vi "Time.Inline Calculate Duration Secs.vi"(8 "Error In Bot":errorcluster, 9 "Start(Sec)":dbl, 11 "Error In Top":errorcluster) -> (0 "Error Out Bot":errorcluster, 1 "Duration(s)":dbl, 3 "Error Out Top":errorcluster)   [LabVIEW 2024, in "EQMF.lvlib" / "Time Utils.lvlib"]
uses:
  Time Utils.lvlib
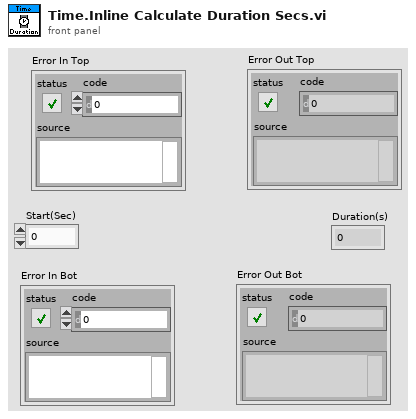
[diagram p1: front panel]
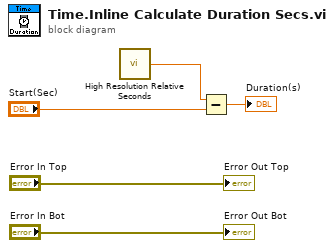
[diagram p0: block diagram]
diagram:
  n1 = call <vilib>:"High Resolution Relative Seconds.vi"() -> ("relative seconds"=w5:dbl)
  n2 = Subtract(x=w5, y="Start(Sec)") -> (x-y=→"Duration(s)":dbl)
  "Error Out Top" <- "Error In Top"
  "Error Out Bot" <- "Error In Bot"
